vi "Bounding Rectangle of Particles.vi"() -> ()   [LabVIEW 2011]
panel:
  in  "Particle Reports (Pixels)":T1(array[cluster]) {"Orientation" format="%.2f"; "Dimensions"."Height" format="%.2f"; "Dimensions"."Width" format="%.2f"; "Center of Mass"."Y" format="%.2f"; "Center of Mass"."X" format="%.2f"; "Bounding Rect"."Bottom" format="%.2f"; "Bounding Rect"."Right" format="%.2f"; "Bounding Rect"."Top" format="%.2f"; "Bounding Rect"."Left" format="%.2f"; "Number of Holes" format="%.2f"; "Area" format="%.2f"}
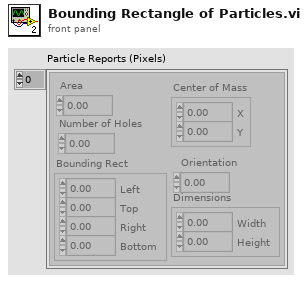
[diagram p1: front panel]
types:
  T1 = cluster{"Area":dbl, "Number of Holes":dbl, "Bounding Rect":cluster{"Left":dbl, "Top":dbl, "Right":dbl, "Bottom":dbl}, "Center of Mass":cluster{"X":dbl, "Y":dbl}, "Orientation":dbl, "Dimensions":cluster{"Width":dbl, "Height":dbl}}[]
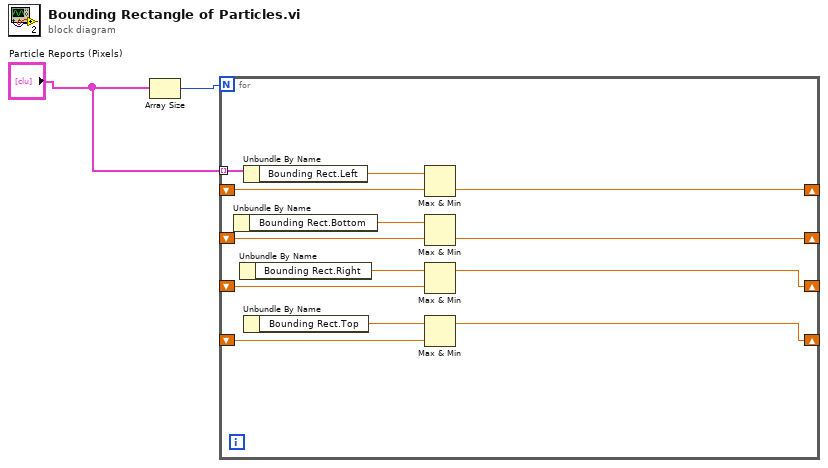
[diagram p0: block diagram]
diagram:
  n1 = Array Size(array="Particle Reports (Pixels)") -> (size(s)=w2:i32)
  n2 = for {
    N: w2 -> [_]
    tunnel: "Particle Reports (Pixels)" -> [w15] mode=indexing
    shift-right: [w13] -> _
    shift-left: _ -> [w12]
    shift-right: [w10] -> _
    shift-left: _ -> [w9]
    shift-right: [w6] -> _
    shift-left: _ -> [w7]
    shift-right: [w4] -> _
    shift-left: _ -> [w3]
    n3 = Unbundle By Name() -> ("Bounding Rect.Bottom"=w11:dbl)  [unwired: 1 in]
    n4 = Unbundle By Name() -> ("Bounding Rect.Right"=w8:dbl)  [unwired: 1 in]
    n5 = Unbundle By Name(w15) -> ("Bounding Rect.Left"=w14:dbl)
    n6 = Unbundle By Name() -> ("Bounding Rect.Top"=w5:dbl)  [unwired: 1 in]
    n7 = Max & Min(x=w14, y=w12) -> (min(x,y)=w13:dbl)  [unwired: 1 out]
    n8 = Max & Min(x=w11, y=w9) -> (min(x,y)=w10:dbl)  [unwired: 1 out]
    n9 = Max & Min(x=w8, y=w7) -> (max(x,y)=w6:dbl)  [unwired: 1 out]
    n10 = Max & Min(x=w5, y=w3) -> (max(x,y)=w4:dbl)  [unwired: 1 out]
  }
